vi "Create Table.vi"() -> ()   [LabVIEW 2019]
uses:
  <vilib>/addons/database/Auxilliary.llb/DB Tools Column Info.ctl
  <vilib>/addons/database/Auxilliary.llb/DB Tools DataTypes.ctl
  <vilib>/addons/database/Connection.llb/DB Tools Open Connec (String).vi
  <vilib>/addons/database/NI_Database_API.lvlib
panel:
  in  "error in (no error)":errorcluster
  in  "Database Name":string="789"
  in  "table":string="Data1"
  in  "column information":T1[](array[typedef])=[{"column name"="ID", "data type"=enum."String", "size"=10, "allow null?"=TRUE}, {"column name"="Grade", "data type"=enum."Double (DBL)", "size"=0, "allow null?"=TRUE}, {"column name"="velocity", "data type"=enum."Double (DBL)", "size"=0, "allow null?"=TRUE}]
  out "error out":errorcluster
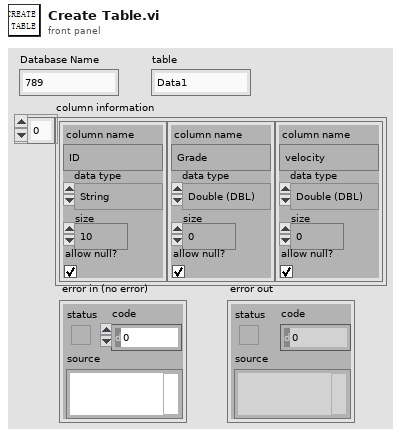
[diagram p1: front panel]
types:
  T1 = typedef "NI_Database_API.lvlib/DB Tools Column Info.ctl" = cluster{"column name":string, "data type":T2, "size":i32, "allow null?":bool}
  T2 = typedef "NI_Database_API.lvlib/DB Tools DataTypes.ctl" = enum16{"String", "Long (I32)", "Single (SGL)", "Double (DBL)", "Date/Time", "Binary"}
  T3 = typedef "NI_Database_API.lvlib/Conn ObjectReference.ctl" = refnum<k1>
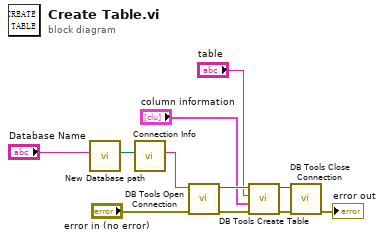
[diagram p0: block diagram]
diagram:
  n1 = call "New Database path.vi"("Database Name"="Database Name") -> ("Database path"=w11:path)  [unwired: 10 in]
  n2 = call "Connection Info.vi"("路径"=w11) -> ("Connection Info"=w9:string)  [unwired: 10 in]
  n3 = call-poly <vilib>:"DB Tools Open Connection.vi"("error in (no error)"="error in (no error)", "connection information"=w9) -> ("error out"=w6:errorcluster, "connection reference"=w7:T3)  [unwired: 6 in]
  n4 = call <vilib>:"DB Tools Create Table.vi"("error in (no error)"=w6, "column information"="column information", "table"="table", "connection reference"=w7) -> ("error out"=w5:errorcluster, "connection reference out"=w4:T3)  [unwired: 4 in]
  n5 = call <vilib>:"DB Tools Close Connection.vi"("error in (no error)"=w5, "connection reference"=w4) -> ("error out"=→"error out":errorcluster)  [unwired: 5 in]
